vi "mouse down action.vi"(8 "engine":refnum<data-value>, 10 "CtlRef":refnum<vi>, 11 "module editor reference":refnum<data-value>) -> (0 "error out":errorcluster)   [LabVIEW 2013, in "My Awesome Control Modules editor node.lvclass"]
uses:
  My Awesome Control Modules editor node.lvclass
  <vilib>/NI/Tag Bus Data Framework/control module/configuration/control module configuration.lvclass
  <vilib>/NI/Tag Bus/tag/tag descriptor.lvclass
  <vilib>/NI/Configuration Framework/serializable configuration/NISE_CEF_serializable configuration.lvclass
  <vilib>/NI/Module Execution Interface/Engine Configuration/engine configuration.lvclass
  <vilib>/NI/Tag Bus Data Framework/Configuration Editor/Classes/Engine Parent/Engine Parent Editor Node.lvclass
  <vilib>/NI/Tag Bus Data Framework/control module/editor node/control module editor.lvclass
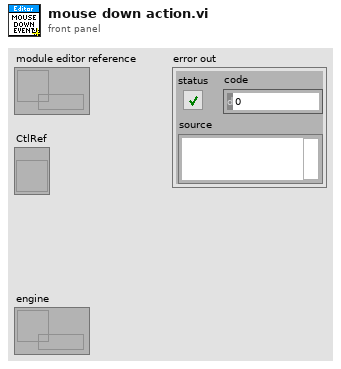
[diagram p1: front panel]
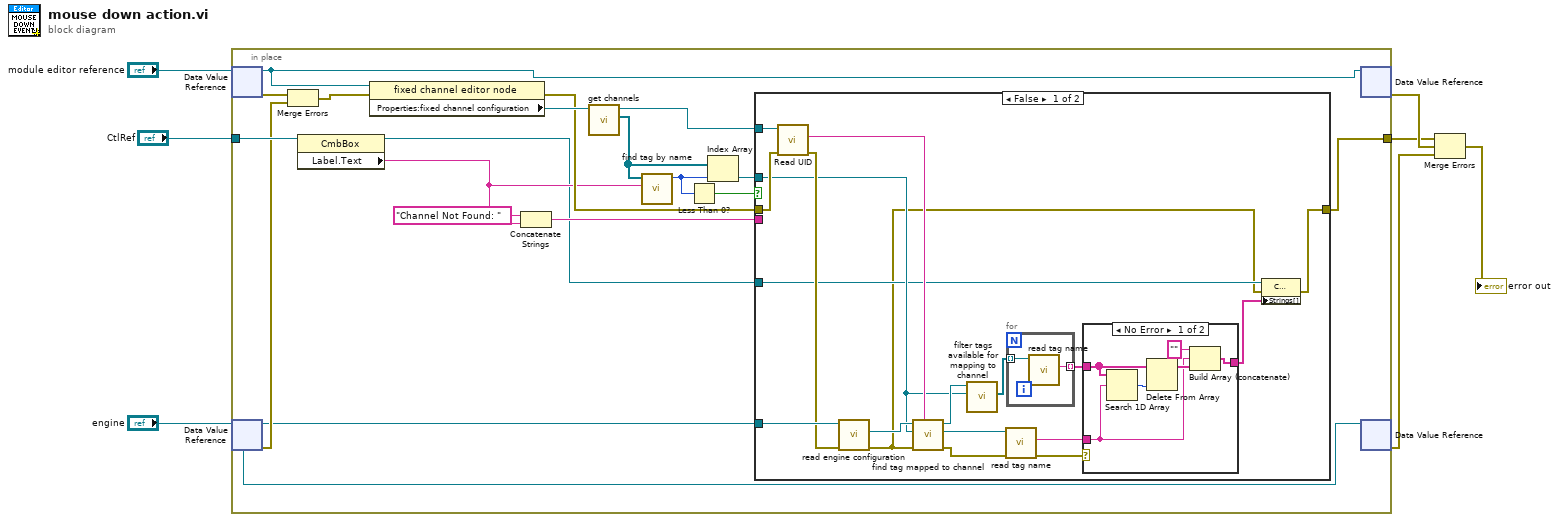
[diagram p0: block diagram]
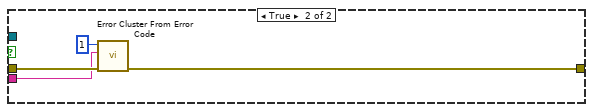
[diagram p3: hidden frame]
diagram:
  n1 = in-place {
    in-place-border: [w20] -> w2
    in-place-border: "CtlRef" -> [w18]
    n2 = in-place-dvr #1("module editor reference") -> (w10:refnum<class "control module editor.lvclass">, w25:errorcluster)
    n3 = in-place-dvr #2("engine") -> (w9:refnum<class "Engine Parent Editor Node.lvclass">, w12:errorcluster)
    n4 = Merge Errors(w25, w12) -> (w13:errorcluster)
    n5 = property class="CmbBox"(reference=w18) -> (reference out=w8:refnum<vi>, "Label.Text"=w17:string)  [unwired: 1 in, 1 out]
    n6 = property class="fixed channel editor node"(reference=w10, error in=w13) -> (error out=w19:errorcluster, "Properties:fixed channel configuration"=w24:refnum<class "control module configuration.lvclass">)  [unwired: 1 out]
    n7 = Concatenate Strings("Channel Not Found: " ("string"), w17) -> (w15:string)
    n8 = call-dynamic "get channels.vi"("fixed channel configuration in"=w24) -> ("channels"=w23:refnum<class "TBM channel.lvclass">[], "fixed channel configuration out"=w11:refnum<class "control module configuration.lvclass">)  [unwired: 9 in]
    n9 = call <vilib>:"find tag by name.vi"("name"=w17, "tags in"=w23) -> ("index"=w22:i32)  [unwired: 9 in]
    n10 = Less Than 0?(x=w22) -> (x < 0?=w21:bool)
    n11 = Index Array(array=w23, index=w22) -> (element=w14:refnum<class "TBM channel.lvclass">)
    n12 = case shown="False" w21 {
      tunnel: [w26 w55] -> w20
      tunnel: w19 -> [w42 w54]
      tunnel: w15 -> [_ w53]
      tunnel: w14 -> [w36 _]
      tunnel: w11 -> [w43 _]
      tunnel: w9 -> [w39 _]
      tunnel: w8 -> [w29 _]
      frame False {
        n13 = call <vilib>:"Read UID.vi"("error in"=w42, "configuration in"=w43) -> ("error out"=w38:errorcluster, "instance id"=w40:string)  [unwired: 7 in, 1 out]
        n14 = call <vilib>:"read engine configuration.vi"("error in"=w38, "Engine Parent Editor Node in"=w39) -> ("error out"=w27:errorcluster, "engine configuration"=w37:refnum<class "engine configuration.lvclass">)  [unwired: 7 in, 1 out]
        n15 = call <vilib>:"find tag mapped to channel.vi"("owner"=w40, "error in"=w27, "channel"=w36, "engine configuration in"=w37) -> ("error out"=w33:errorcluster, "tag"=w34:refnum<class "tag descriptor.lvclass">, "engine configuration out"=w41:refnum<class "engine configuration.lvclass">)  [unwired: 5 in]
        n16 = call <vilib>:"filter tags available for mapping to channel.vi"("channel to map to"=w36, "engine configuration in"=w41) -> ("filtered tags"=w35:refnum<class "tag descriptor.lvclass">[])  [unwired: 8 in, 1 out]
        n17 = call <vilib>:"read tag name.vi"("error in"=w33, "system tag in"=w34) -> ("error out"=w32:errorcluster, "name"=w30:string)  [unwired: 7 in, 1 out]
        n18 = for {
          tunnel: w35 -> [w45] mode=indexing
          tunnel: [w44] -> w31 mode=indexing
          n19 = call <vilib>:"read tag name.vi"("system tag in"=w45) -> ("name"=w44:string)  [unwired: 8 in, 2 out]
        }
        n20 = case shown="No Error" w32 {
          tunnel: w31 -> [w50 w52]
          tunnel: [w47 w52] -> w28
          tunnel: w30 -> [w48 _]
          frame No Error {
            n21 = Search 1D Array(1D array=w50, element=w48) -> (index of element=w51:i32)  [unwired: 1 in]
            n22 = Delete From Array(array=w50, index=w51) -> (array with subset deleted=w49:string[])  [unwired: 1 in, 1 out]
            n23 = Build Array (concatenate)("" ("element"), w48, w49) -> (w47:string[])
          }
          frame Error {
          }
        }
        n24 = property class="CmbBox"(reference=w29, error in=w27, "Strings[]"=w28) -> (error out=w26:errorcluster)  [unwired: 1 out]
      }
      frame True {
        n25 = call <vilib>:"Error Cluster From Error Code.vi"("error in (no error)"=w54, "error message (\"\")"=w53, "error code (0)"=1) -> ("error out"=w55:errorcluster)  [unwired: 6 in]
      }
    }
    n26 = in-place-dvr #1(w10) -> (w3:errorcluster)  [unwired: 1 out]
    n27 = in-place-dvr #2(w9) -> (w6:errorcluster)  [unwired: 1 out]
  }
  n28 = Merge Errors(w2, w3, w6) -> (→"error out":errorcluster)
